vi "CircularBuffer.ReftoDVR.vi"(10 "Ref":u32 format="%08x") -> (2 "Ref":T1)   [LabVIEW 2013, in "CircularBuffer.lvclass"]
doc: "JKI State Machine Objects (SMO) 1.0.0.5\nJKI - JKI\nCopyright (c) 2016, JKI"
uses:
  CircularBuffer.lvclass
  Typedefs/ValueChanged--EventData--Cluster.ctl
  Typedefs/PublicEvents--Cluster.ctl
  Typedefs/NewBufferSize--Cluster.ctl
  Typedefs/ProtectedEvents--Cluster.ctl
  Typedefs/PrivateData--Cluster.ctl
  Typedefs/PrivateData--Ref.ctl
  Typedefs/PrivateEvents--Cluster.ctl
  Typedefs/PrivateEvents--CircularBuffer.GetElement.ctl
  types/type/type.lvclass
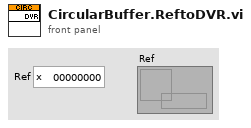
[diagram p1: front panel]
types:
  T1 = typedef "CircularBuffer.lvclass/PrivateData--Ref.ctl" = refnum<data-value>
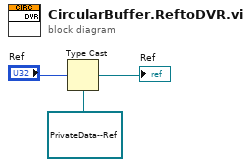
[diagram p0: block diagram]
diagram:
  n1 = Type Cast(type=T1 refnum ("Ref"), x="Ref") -> (*(type *) &x=→"Ref":T1)
